vi "Adquisicio_projecte_InsEl.vi"() -> ()   [LabVIEW 2014]
uses:
  <vilib>/DAQmx/create/channels.llb/DAQmx Create Channel (AI-Voltage-Basic).vi
  <vilib>/DAQmx/configure/timing.llb/DAQmx Timing (Sample Clock).vi
  <vilib>/DAQmx/read.llb/DAQmx Read.vi
  <vilib>/DAQmx/read.llb/DAQmx Read (Analog 1D Wfm NChan NSamp).vi
  <vilib>/addons/Multicore Analysis and Sparse Matrix/Statistics/_statistics/Mean (DBL).vi
  <vilib>/addons/Multicore Analysis and Sparse Matrix/Statistics/NI_MASM_Statistics.lvlib
panel:
  out "Numeric 5":dbl
  out "Numeric 4":dbl
  out "Numeric 3":dbl
  out "Numeric 2":dbl
  out "Array":dbl[][](array[numeric])
  in  "?":bool
  in  "nº mitjana":dbl
  in  "Durada adquisició":dbl
  in  "Temps entre adquisicions":dbl
  in  "Canals":i8(slide) scale=1.0..4.0
  in  "?":bool
  out "data":waveform(dbl)[](graph)
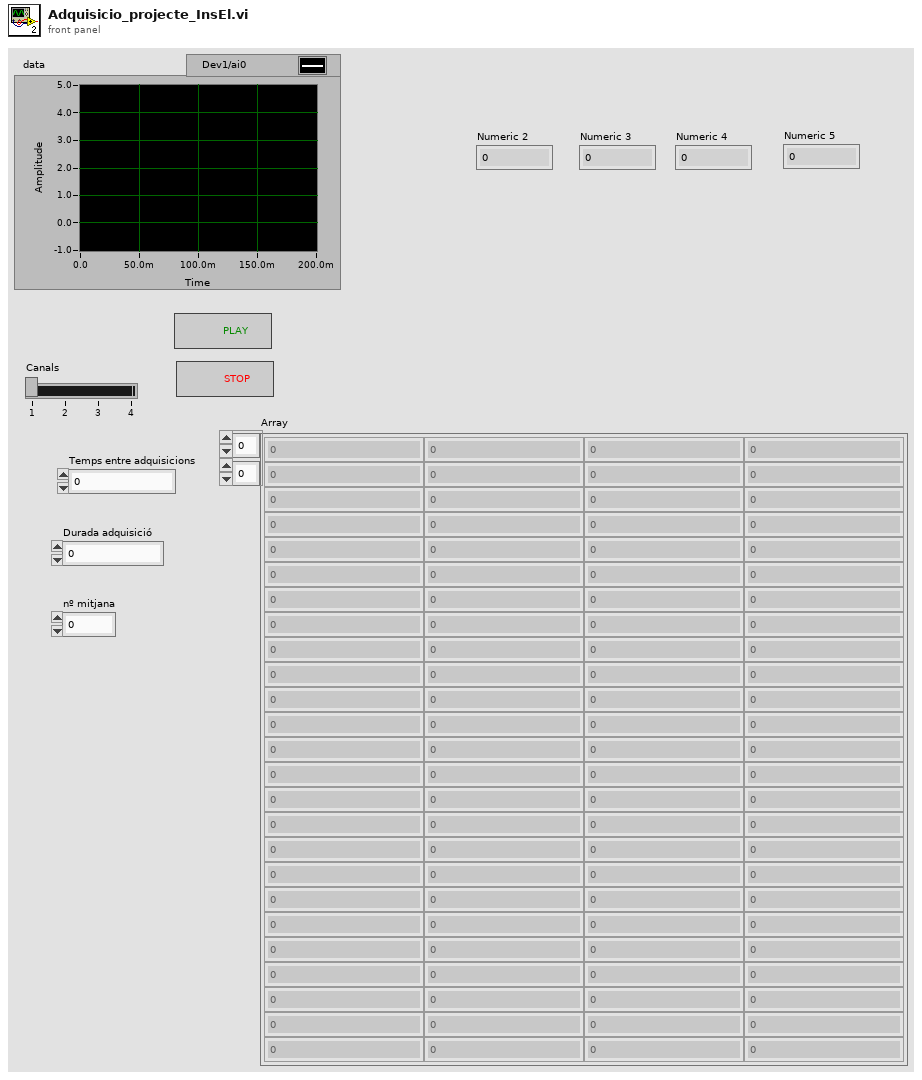
[diagram p1: front panel]
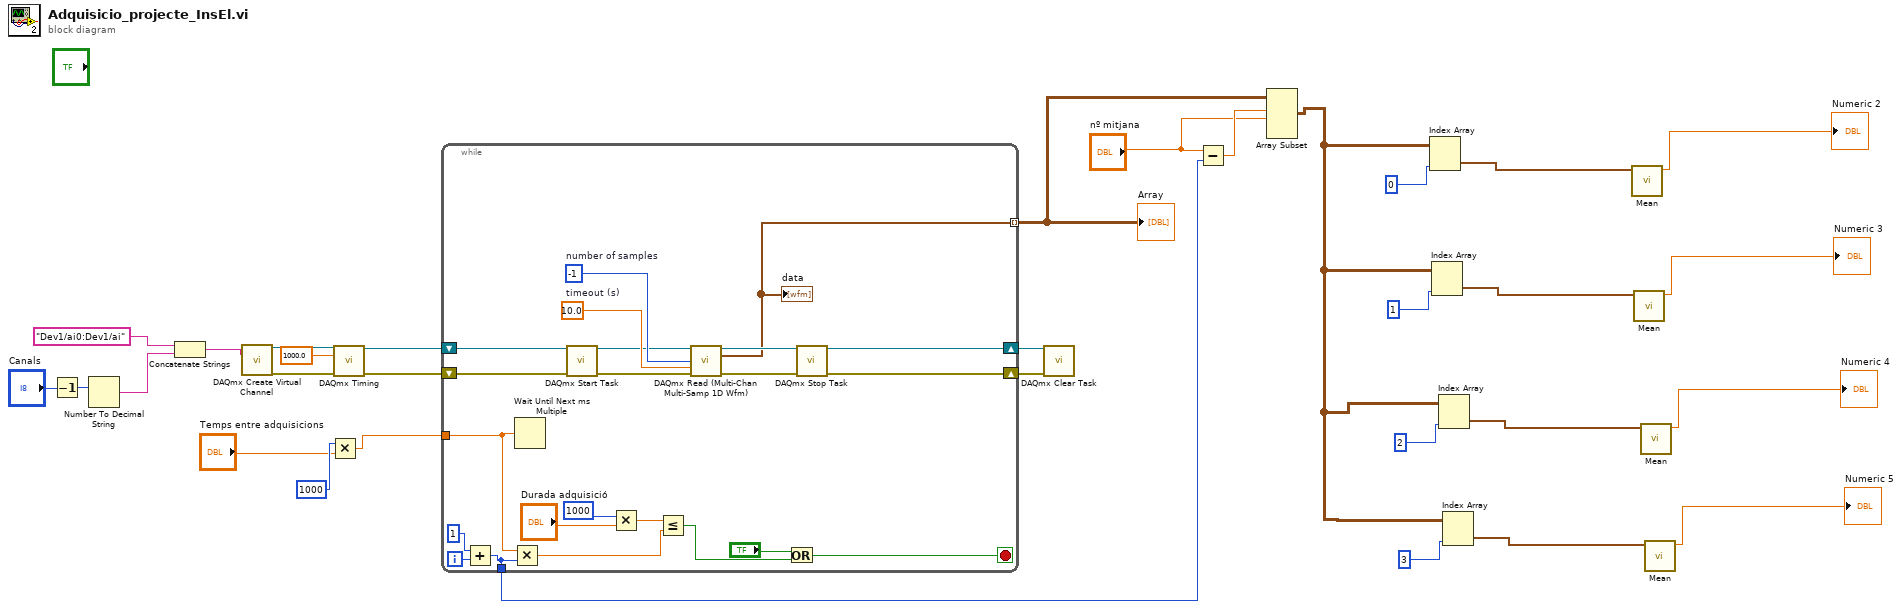
[diagram p0: block diagram]
diagram:
  n1 = Decrement(x="Canals") -> (x-1=w21:i8)
  n2 = Number To Decimal String(number=w21) -> (decimal integer string=w23:string)  [unwired: 1 in]
  n3 = Concatenate Strings "Concatenate Strings"("Dev1/ai0:Dev1/ai", w23) -> (w25:string)
  n4 = call-poly <vilib>:"DAQmx Create Virtual Channel.vi"("physical channels"=w25) -> ("task out"=w27:refnum<k21>, "error out"=w28:errorcluster)  [unwired: 13 in]
  n5 = Multiply(x=1000, y="Temps entre adquisicions") -> (x*y=w18:dbl)
  n6 = call-poly <vilib>:"DAQmx Timing.vi"("task/channels in"=w27, "rate"=1000.0, "error in"=w28) -> ("task out"=w30:refnum<k21>, "error out"=w29:errorcluster)  [unwired: 11 in]
  n7 = while {
    shift-right: [w50] -> w32
    shift-left: w30 -> [w46]
    shift-right: [w49] -> w31
    shift-left: w29 -> [w45]
    tunnel: w18 -> [w36]
    tunnel: [w33] -> w17 mode=indexing
    tunnel: [w34] -> w16
    i -> [w37]
    stop <- w44 stop-if-true
    w53 = 10.0  # timeout (s)
    w54 = -1  # number of samples
    n8 = Add(x=1, y=w37) -> (x+y=w34:i32)
    n9 = Multiply(x=w36, y=w34) -> (x*y=w38:dbl)
    n10 = Wait Until Next ms Multiple(millisecond multiple=w36) -> ()  [unwired: 1 out]
    n11 = call <vilib>:"DAQmx Start Task.vi"("task/channels in"=w46, "error in"=w45) -> ("task out"=w51:refnum<k21>, "error out"=w52:errorcluster)  [unwired: 12 in]
    n12 = Multiply(x=1000, y="Durada adquisició") -> (x*y=w40:dbl)
    n13 = Less Or Equal?(x=w40, y=w38) -> (x <= y?=w39:bool)
    n14 = call-poly "DAQmx Read (Multi-Chan Multi-Samp 1D Wfm).vi"("task/channels in"=w51, "number of samples per channel"=w54, "timeout"=w53, "error in"=w52) -> ("task out"=w48:refnum<k21>, "data"=w33:waveform(dbl)[], "error out"=w47:errorcluster)  [unwired: 9 in]
    "data" <- w33
    n15 = Or(x="?", y=w39) -> (x .or. y?=w44:bool)
    n16 = call <vilib>:"DAQmx Stop Task.vi"("task/channels in"=w48, "error in"=w47) -> ("task out"=w50:refnum<k21>, "error out"=w49:errorcluster)  [unwired: 12 in]
  }
  "Array" <- w17
  n17 = call <vilib>:"DAQmx Clear Task.vi"("task in"=w32, "error in"=w31) -> ()  [unwired: 13 in, 1 out]
  n18 = Subtract(x="nº mitjana", y=w16) -> (x-y=w15:dbl)
  n19 = Array Subset(array=w17, index (row)=w15, length (row)="nº mitjana") -> (w1:waveform(dbl)[][])  [unwired: 2 in]
  n20 = Index Array(array=w1, index (col)=0 ("disabled index (col)")) -> (element=w12:waveform(dbl)[])  [unwired: 1 in]
  n21 = Index Array(array=w1, index (col)=1 ("disabled index (col)")) -> (element=w9:waveform(dbl)[])  [unwired: 1 in]
  n22 = Index Array(array=w1, index (col)=2 ("disabled index (col)")) -> (element=w6:waveform(dbl)[])  [unwired: 1 in]
  n23 = Index Array(array=w1, index (col)=3 ("disabled index (col)")) -> (element=w3:waveform(dbl)[])  [unwired: 1 in]
  n24 = call-poly <vilib>:"Mean.vi"("X"=w12) -> ("mean"=→"Numeric 2":dbl)  [unwired: 9 in, 1 out]
  n25 = call-poly <vilib>:"Mean.vi"("X"=w9) -> ("mean"=→"Numeric 3":dbl)  [unwired: 9 in, 1 out]
  n26 = call-poly <vilib>:"Mean.vi"("X"=w6) -> ("mean"=→"Numeric 4":dbl)  [unwired: 9 in, 1 out]
  n27 = call-poly <vilib>:"Mean.vi"("X"=w3) -> ("mean"=→"Numeric 5":dbl)  [unwired: 9 in, 1 out]
